vi "spectral measurements and concatination of a signals.vi"() -> ()   [LabVIEW 2025]
uses:
  <vilib>/express/express analysis/Spectral/Block/exnSpectralBlock spectral measurements power poly.vi
  <vilib>/express/express analysis/Spectral/Block/exnSpectralBlock spectral measurements power DDT.vi
  <vilib>/express/express analysis/Spectral/XNode/ExpressSpectralMeasurementsBlockNode.xnode
panel:
  out "FFT PEAK MUL":dynamicdata(graph)
  out "FFT PEAK SUB":dynamicdata(graph)
  out "FFT PEAK ADDTION":dynamicdata(graph)
  out "mutliplication of signal":dynamicdata(graph)
  out "subtraction of signal":dynamicdata(graph)
  out "addtion of singnal":dynamicdata(graph)
  out "signal 2":dynamicdata(graph) caption="Sine"
  out "singnal 1":dynamicdata(graph) caption="Sine"
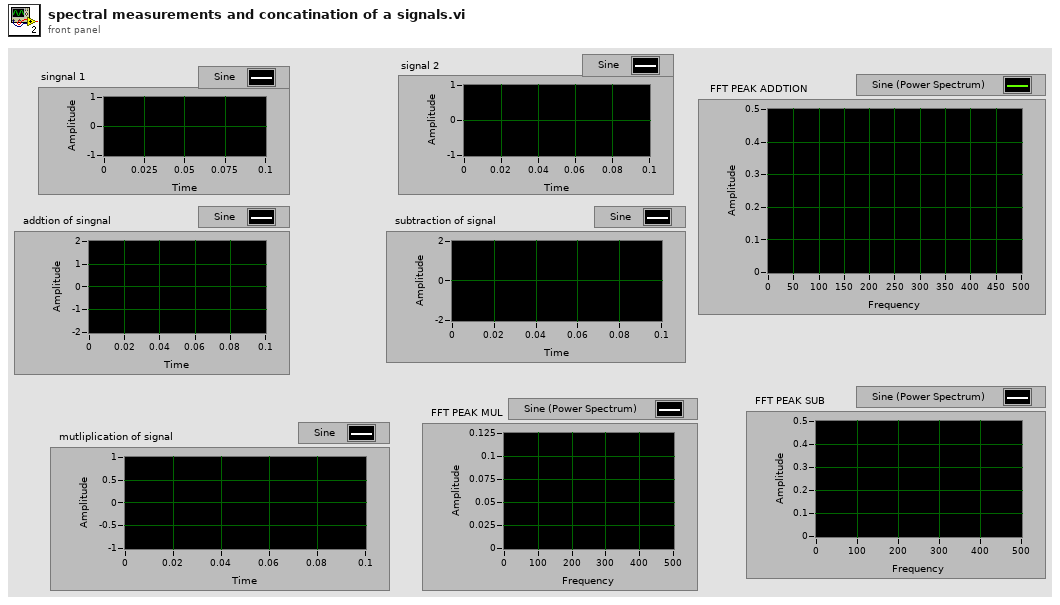
[diagram p1: front panel]
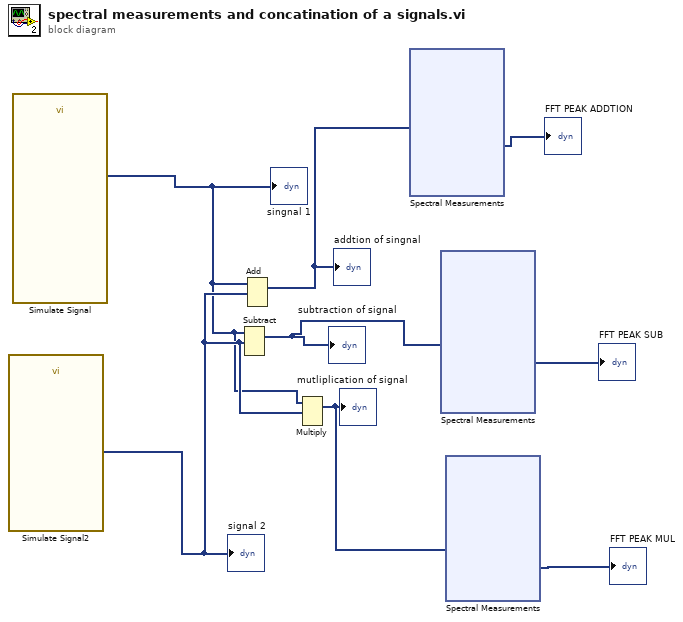
[diagram p0: block diagram]
diagram:
  n1 = call "Simulate Signal2"() -> ("Sine"=w8:dynamicdata)  [unwired: 14 in, 1 out]
  "signal 2" <- w8
  n2 = call "Simulate Signal"() -> ("Sine"=w7:dynamicdata)  [unwired: 14 in, 1 out]
  "singnal 1" <- w7
  n3 = Subtract(1:w8, 2:w7) -> (0:w4:dynamicdata)  [unwired: 1 in, 1 out]
  "subtraction of signal" <- w4
  n4 = Add(1:w8, 2:w7) -> (0:w6:dynamicdata)  [unwired: 1 in, 1 out]
  "addtion of singnal" <- w6
  n5 = Multiply(1:w8, 2:w7) -> (0:w2:dynamicdata)  [unwired: 1 in, 1 out]
  "mutliplication of signal" <- w2
  n6 = xnode "Spectral Measurements"("Signals"=w6) -> ("Power Spectrum"=→"FFT PEAK ADDTION":dynamicdata)  [unwired: 1 in, 1 out]
  n7 = xnode "Spectral Measurements"("Signals"=w4) -> ("Power Spectrum"=→"FFT PEAK SUB":dynamicdata)  [unwired: 1 in, 1 out]
  n8 = xnode "Spectral Measurements"("Signals"=w2) -> ("Power Spectrum"=→"FFT PEAK MUL":dynamicdata)  [unwired: 1 in, 1 out]
